vi "Item History.vi"(11 "reference in":T1) -> (3 "reference out":T1)   [LabVIEW 2016]
uses:
  Control/State machine.ctl
  <vilib>/Utility/miscctls.llb/LVPointTypeDef.ctl
  <vilib>/addons/database/NI_Database_API.lvlib
  <vilib>/addons/database/Recordset.llb/Rec Fetch Recordset Data (R).vi
  <vilib>/addons/database/Recordset.llb/Rec Destroy - Connection.vi
  <vilib>/addons/database/Connection.llb/Conn Execute.vi
  <vilib>/addons/database/_DB Variant To Data/Database Variant To Data.xnode
  <vilib>/Utility/miscctls.llb/LVRowAndColumnUnsignedTypeDef.ctl
  <vilib>/addons/database/Connection.llb/DB Tools Open Connec (Path).vi
  <vilib>/addons/database/Connection.llb/Conn ObjectReference.ctl
panel:
  in  "Sort data":string[][](array[string])
  in  "Mode":bool=TRUE
  in  "Stock":string
  in  "Location":string
  in  "Lot Size":string
  in  "Maker":string
  in  "Part Name":string
  in  "Part No.":string
  in  "Product":string
  in  "Select Month":timestamp format="%<%d/%m/%Y>T"
  in  "Item Code":string(combo)
  out "Table":string[][](table)
  # "ITEM HISTORY"
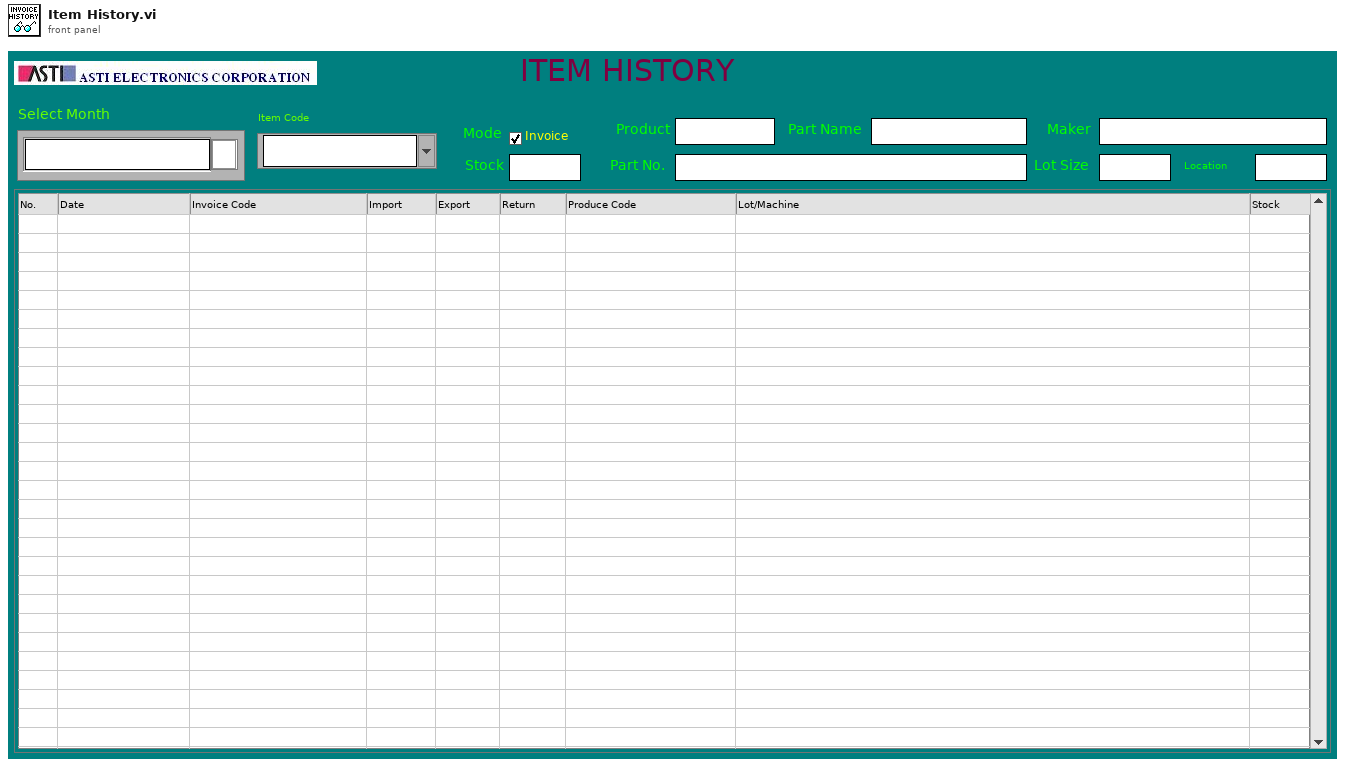
[diagram p1: front panel]
types:
  T1 = typedef "NI_Database_API.lvlib/Conn ObjectReference.ctl" = refnum<k1>
  T2 = typedef "LVPointTypeDef.ctl" = cluster{"Horizontal":i16, "Vertical":i16}
  T3 = typedef "State machine.ctl" = enum16{"Licence check", "Initial", "Log in", "Creat Config file", "Network setting", "Creat database 1", "Creat database 2", "Creat database 3", "Transfer", "Begin", "Exit"}
  T4 = typedef "LVRowAndColumnUnsignedTypeDef.ctl" = cluster{"Row":u32, "Column":u32}
  T5 = typedef "NI_Database_API.lvlib/Rec ObjectReference.ctl" = refnum<k1>
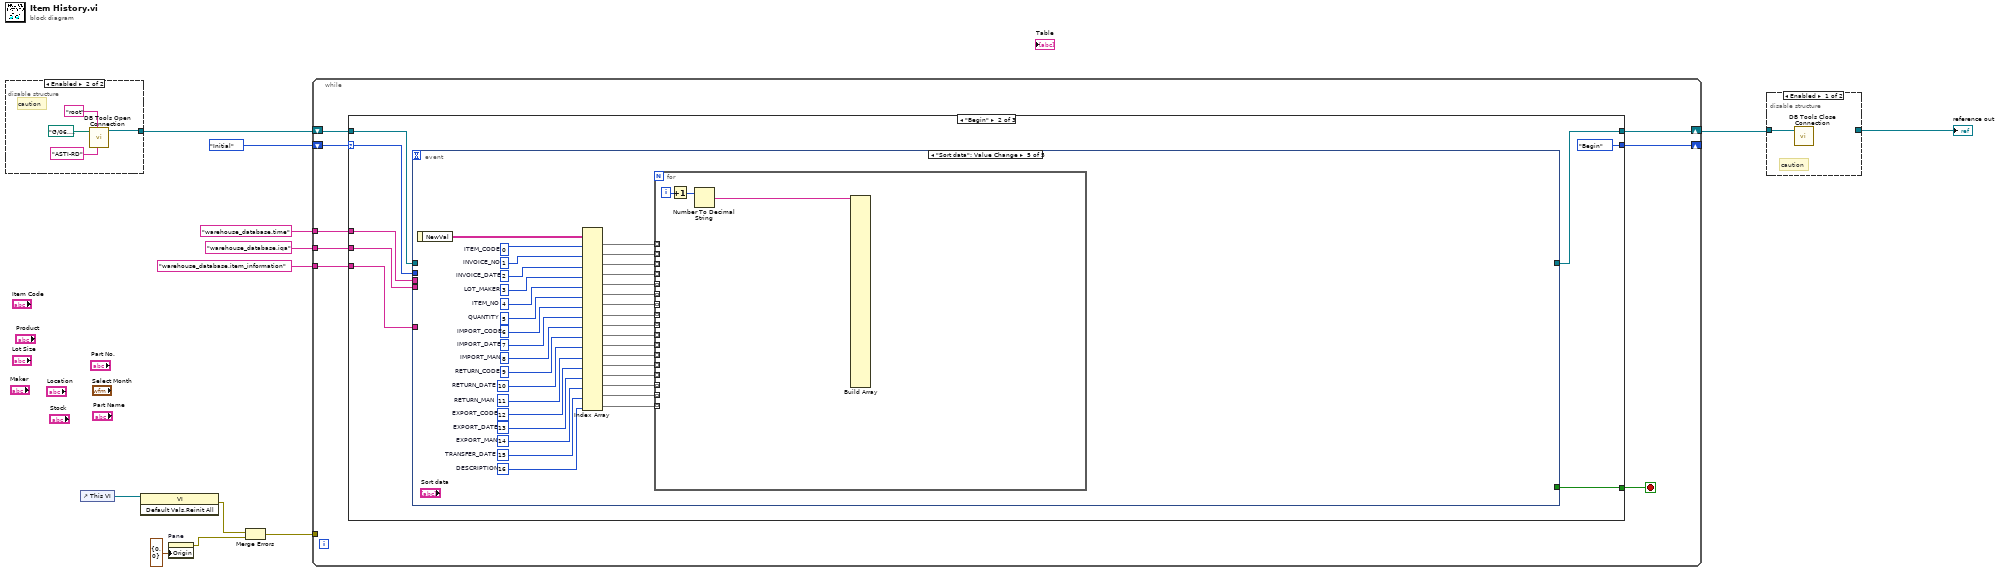
[diagram p0: block diagram]
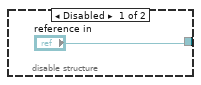
[diagram p3: hidden frame]
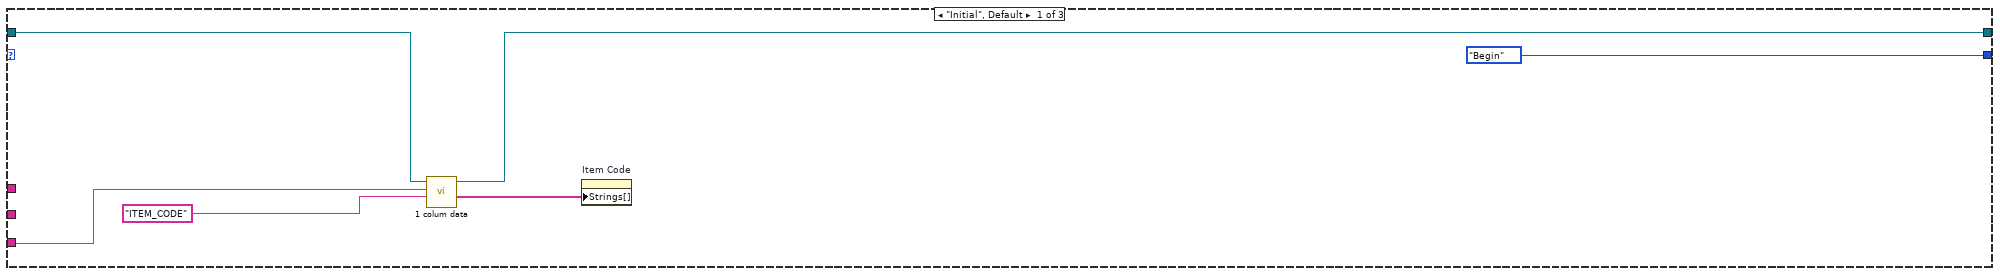
[diagram p4: hidden frame]
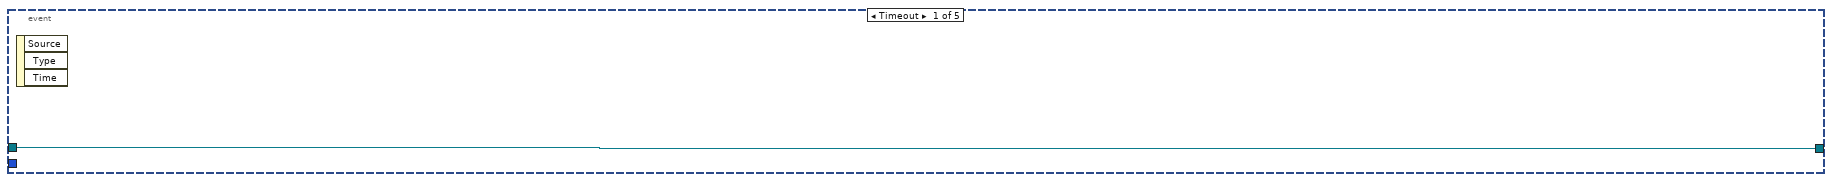
[diagram p5: hidden frame]
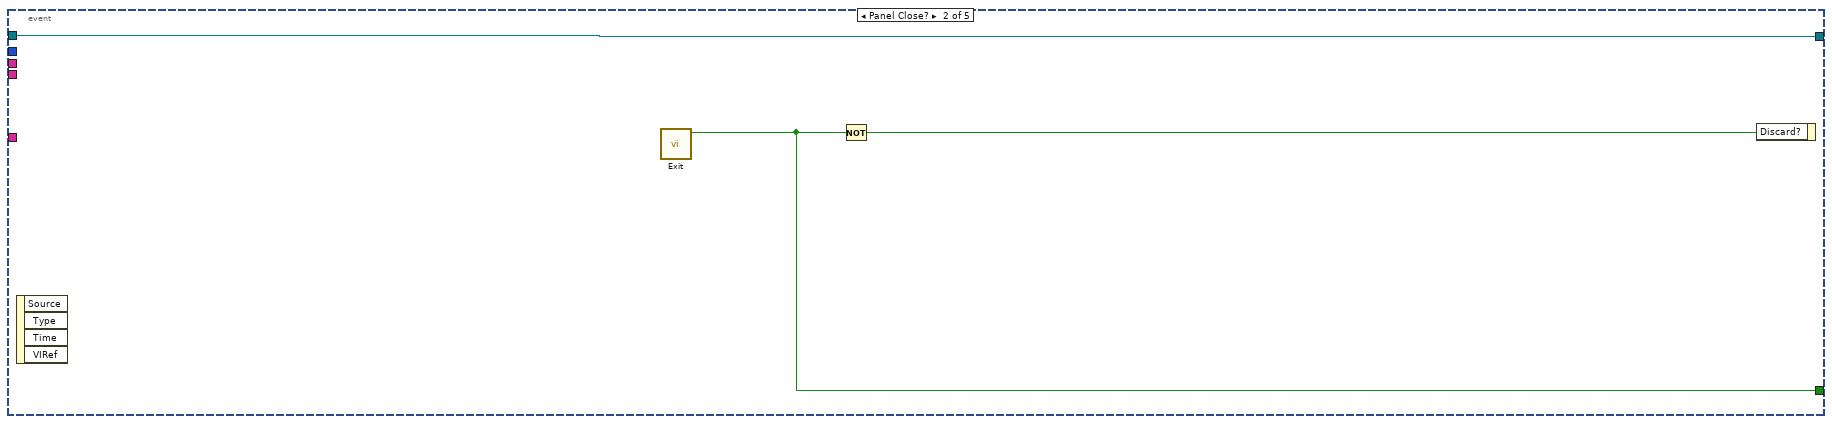
[diagram p6: hidden frame]
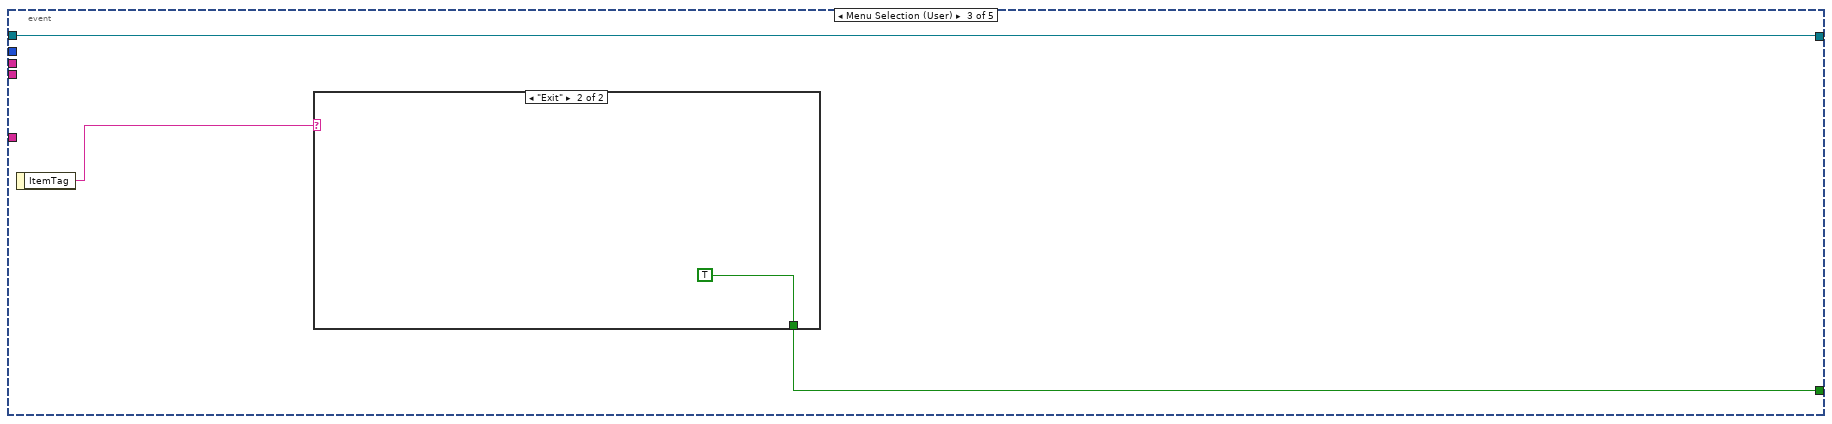
[diagram p7: hidden frame]
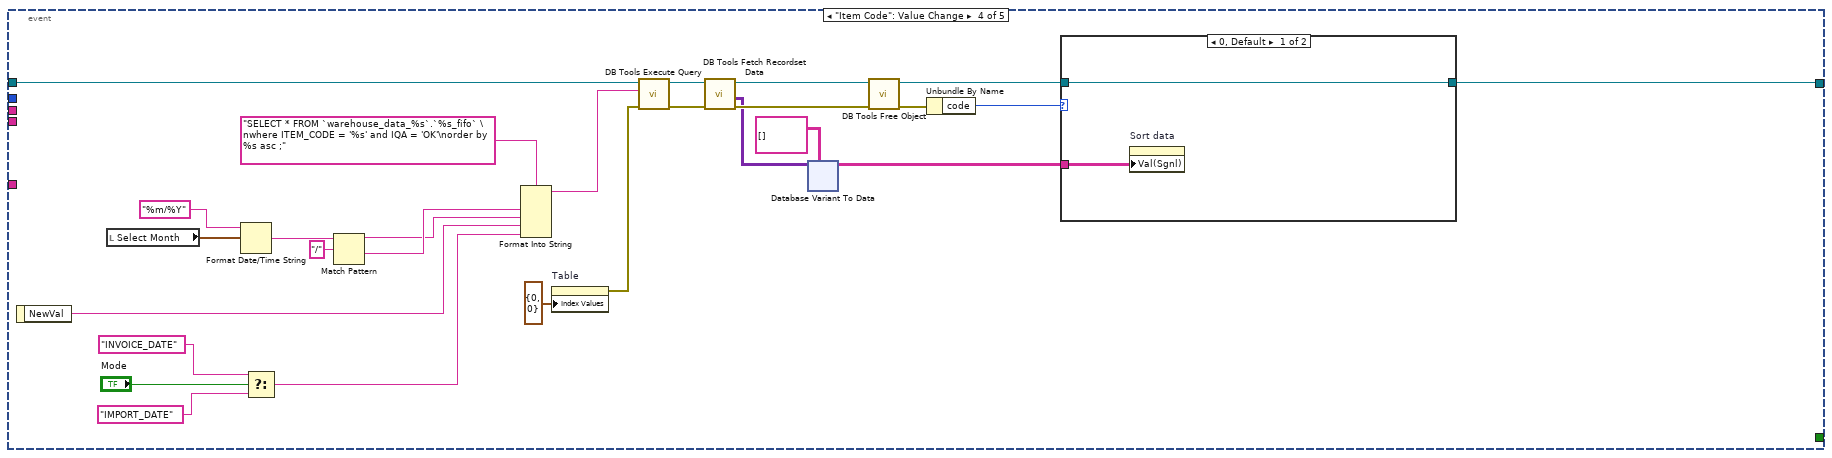
[diagram p9: hidden frame]
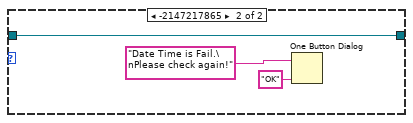
[diagram p10: hidden frame]
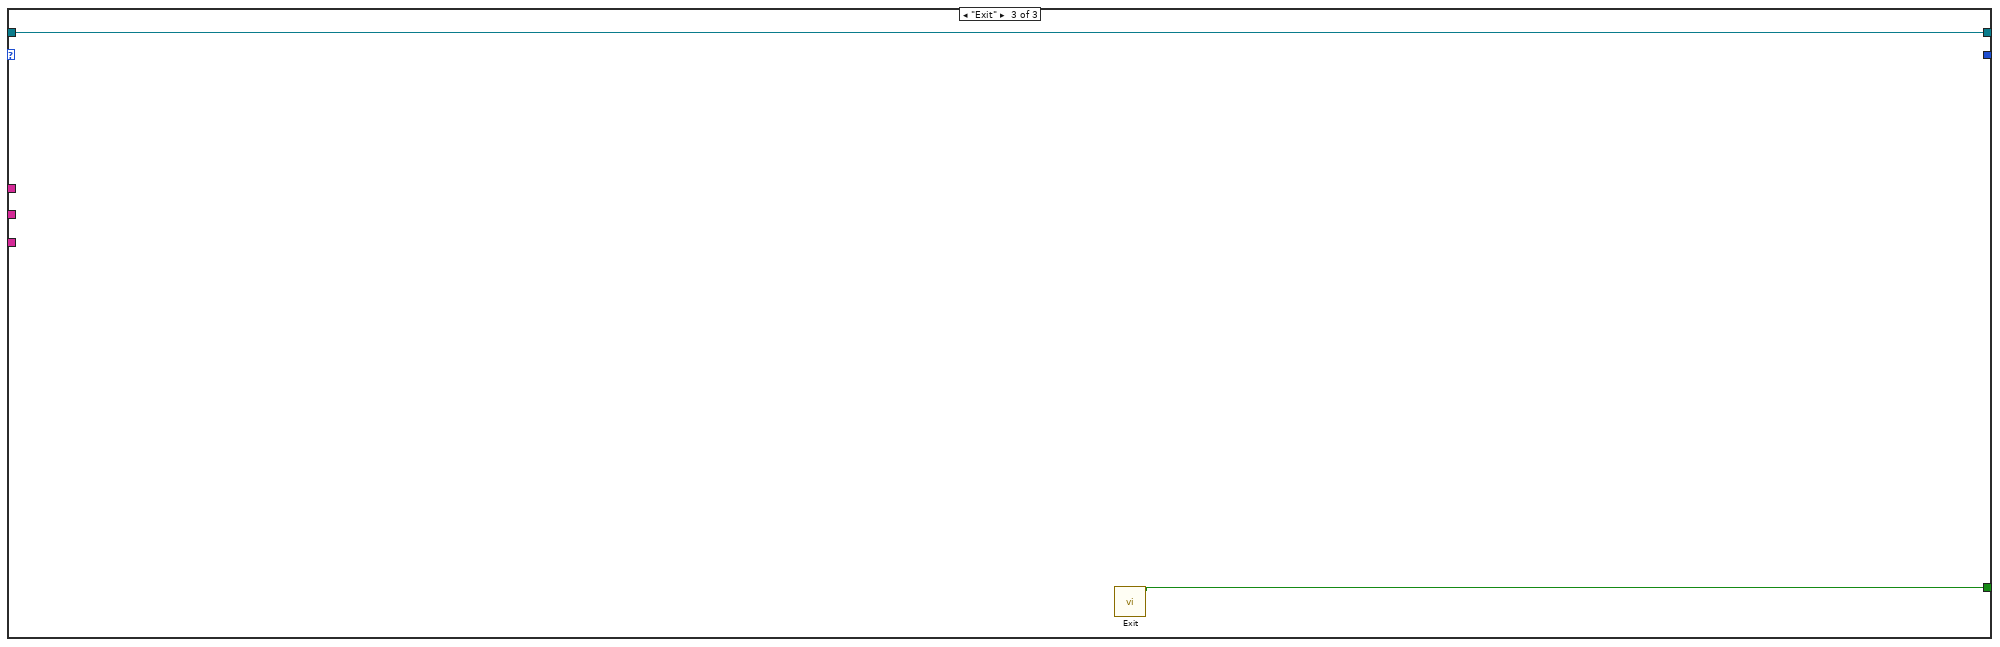
[diagram p11: hidden frame]
diagram:
  n1 = disable-structure shown="Enabled" {
    disable-tunnel: ["reference in" w17] -> w3
    frame Disabled {
    }
    frame Enabled {
      # "caution"
      n2 = call-poly <vilib>:"DB Tools Open Connection.vi"("password"="ASTI-RD", "userID"="root", "connection information"=path "G:/06. Data/Data/05. AEC/07. New Storage Management/Setting/Database local.dsn") -> ("connection reference"=w17:T1)  [unwired: 5 in, 1 out]
    }
  }
  n3 = control-ref of="This VI"() -> (w11:refnum<vi>)
  n4 = invoke class="VI" method="Default Vals.Reinit All"(reference=w11) -> (error out=w9:errorcluster)  [unwired: 2 in, 2 out]
  n5 = property on="Pane" class="Pane"("Origin"=T2 {"Horizontal"=0, "Vertical"=0}) -> (error out=w8:errorcluster)  [unwired: 2 in, 1 out]
  n6 = Merge Errors(w9, w8) -> (w7:errorcluster)
  n7 = while {
    shift-right: [w23] -> _
    shift-left: State_machine."Initial" ("Enum") -> [w24]
    shift-right: [w22] -> w2
    shift-left: w3 -> [w21]
    tunnel: w7 -> [_]
    tunnel: "warehouse_database.time" ("table") -> [w20]
    tunnel: "warehouse_database.iqa" ("table") -> [w19]
    tunnel: "warehouse_database.item_information" -> [w18]
    stop <- w25 stop-if-true
    n8 = case shown="\"Begin\"" w24 {
      selector: w24 -> [_ w36 _]
      tunnel: [_ w39 w162] -> w25
      tunnel: [State_machine."Begin" ("Enum") State_machine."Begin" ("Enum") _] -> w23
      tunnel: [w29 w37 w163] -> w22
      tunnel: w21 -> [w30 w38 w163]
      tunnel: w20 -> [_ w34 _]
      tunnel: w19 -> [_ w33 _]
      tunnel: w18 -> [w26 w32 _]
      frame "Initial", Default {
        n9 = call "1 colum data.vi"("column"="ITEM_CODE" ("String"), "table"=w26, "Refnum in"=w30) -> ("data"=w27:string[], "Refnum out"=w29:T1)  [unwired: 6 in, 1 out]
        n10 = property on="Item Code" class="CmbBox"("Strings[]"=w27) -> ()  [unwired: 2 in, 2 out]
      }
      frame "Begin" {
        n11 = event shown="[4] \"Sort data\": Value Change" {
          selector: _ -> [_ _ _ _ _]
          dyn-events: _ -> [_ _ _ _ _]
          timeout: _ -> [_ _ _ _ _]
          tunnel: [_ w43 w45 _ _] -> w39
          tunnel: w38 -> [w40 w41 w44 w74 _]
          tunnel: [w40 w41 w44 w55 _] -> w37
          tunnel: w36 -> [_ _ _ _ _]
          tunnel: w34 -> [_ _ _ _ _]
          tunnel: w33 -> [_ _ _ _ _]
          tunnel: w32 -> [_ _ _ _ _]
          event Timeout {
            n12 = event-data() -> ()  [unwired: 1 in, 3 out]
          }
          event Panel Close? {
            n13 = event-data() -> ()  [unwired: 1 in, 4 out]
            n14 = call "Exit.vi"() -> ("T button?"=w43:bool)  [unwired: 11 in]
            n15 = Not(x=w43) -> (.not. x?=w42:bool)
            n16 = event-data("Discard?"=w42) -> ()  [unwired: 1 in, 1 out]
          }
          event Menu Selection (User) {
            n17 = event-data() -> ("ItemTag"=w46:string)  [unwired: 1 in]
            n18 = case shown="\"Exit\"" w46 {
              tunnel: [_ TRUE] -> w45
              frame "False", Default {
              }
              frame "Exit" {
              }
            }
          }
          event "Item Code": Value Change {
            n19 = event-data() -> ("NewVal"=w61:string)  [unwired: 1 in]
            n20 = local read "Select Month"() -> (w69:timestamp)
            n21 = Format Date/Time String(time format string (%c)="%m/%Y", seconds (now)=w69) -> (date/time string=w67:string)  [unwired: 1 in]
            n22 = Select(t="INVOICE_DATE", s="Mode", f="IMPORT_DATE") -> (s? t:f=w51:string)
            n23 = Match Pattern(string=w67, regular expression="/") -> (before substring=w62:string, after substring=w63:string)  [unwired: 1 in, 2 out]
            n24 = Format Into String(format string="SELECT * FROM `warehouse_data_%s`.`%s_fifo` \nwhere ITEM_CODE = '%s' and IQA = 'OK'\norder by %s asc ;", w63, w62, w61, w51) -> (resulting string=w64:string)  [unwired: 2 in, 1 out]
            n25 = property on="Table" class="Tbl (strict)"("Index Values"=T4 {"Row"=0, "Column"=0}) -> (error out=w53:errorcluster)  [unwired: 2 in, 1 out]
            n26 = call-poly <vilib>:"DB Tools Execute Query.vi"("error in (no error)"=w53, "SQL query"=w64, "connection reference"=w74) -> ("error out"=w71:errorcluster, "recordset reference"=w73:T5)  [unwired: 5 in]
            n27 = call-poly <vilib>:"DB Tools Fetch Recordset Data.vi"("error in (no error)"=w71, "recordset reference"=w73) -> ("error out"=w70:errorcluster, "recordset data"=w60:variant[][], "recordset reference out"=w72:T5)  [unwired: 3 in]
            n28 = xnode "Database Variant To Data"("database variant"=w60, "type"=string[][] []) -> ("data"=w48:string[][])  [unwired: 1 in, 1 out]
            n29 = call-poly <vilib>:"DB Tools Free Object.vi"("error in (no error)"=w70, "recordset reference"=w72) -> ("error out"=w58:errorcluster, "connection reference"=w56:T1)  [unwired: 8 in]
            n30 = Unbundle By Name(w58) -> ("code"=w57:i32)
            n31 = case shown="0, Default" w57 {
              tunnel: [w76 w79] -> w55
              tunnel: w56 -> [w76 w79]
              tunnel: w48 -> [w75 _]
              frame 0, Default {
                n32 = property on="Sort data" class="Arr (strict)"("Val(Sgnl)"=w75) -> ()  [unwired: 2 in, 2 out]
              }
              frame -2147217865 {
                n33 = One Button Dialog(message="Date Time is Fail.\nPlease check again!", button name ("OK")="OK") -> ()  [unwired: 1 out]
              }
            }
          }
          event "Sort data": Value Change {
            w141 = 16  # DESCRIPTION
            w142 = 15  # TRANSFER_DATE
            w143 = 14  # EXPORT_MAN
            w144 = 13  # EXPORT_DATE
            w145 = 12  # EXPORT_CODE
            w146 = 11  # RETURN_MAN
            w147 = 10  # RETURN_DATE
            w148 = 9  # RETURN_CODE
            w149 = 8  # IMPORT_MAN
            w150 = 7  # IMPORT_DATE
            w151 = 6  # IMPORT_CODE
            w152 = 5  # QUANTITY
            w153 = 4  # ITEM_NO
            w154 = 3  # LOT_MAKER
            w155 = 2  # INVOICE_DATE
            w156 = 1  # INVOICE_NO
            w157 = 0  # ITEM_CODE
            n34 = event-data() -> ("NewVal"=w158:string[][])  [unwired: 1 in]
            n35 = Index Array(array=w158, index (col) #1=w157, index (col) #2=w156, index (col) #3=w155, index (col) #4=w154, index (col) #5=w153, index (col) #6=w152, index (col) #7=w151, index (col) #8=w150, index (col) #9=w149, index (col) #10=w148, index (col) #11=w147, index (col) #12=w146, index (col) #13=w145, index (col) #14=w144, index (col) #15=w143, index (col) #16=w142, index (col) #17=w141) -> (element #1=w140:string[], element #2=w139:string[], element #3=w138:string[], element #4=w137:string[], element #5=w136:string[], element #6=w135:string[], element #7=w134:string[], element #8=w133:string[], element #9=w132:string[], element #10=w131:string[], element #11=w130:string[], element #12=w129:string[], element #13=w128:string[], element #14=w127:string[], element #15=w126:string[], element #16=w125:string[], element #17=w124:string[])  [unwired: 17 in]
            n36 = for {
              tunnel: w140 -> [_] mode=indexing
              tunnel: w139 -> [_] mode=indexing
              tunnel: w138 -> [_] mode=indexing
              tunnel: w137 -> [_] mode=indexing
              tunnel: w136 -> [_] mode=indexing
              tunnel: w135 -> [_] mode=indexing
              tunnel: w134 -> [_] mode=indexing
              tunnel: w133 -> [_] mode=indexing
              tunnel: w132 -> [_] mode=indexing
              tunnel: w131 -> [_] mode=indexing
              tunnel: w130 -> [_] mode=indexing
              tunnel: w129 -> [_] mode=indexing
              tunnel: w128 -> [_] mode=indexing
              tunnel: w127 -> [_] mode=indexing
              tunnel: w126 -> [_] mode=indexing
              tunnel: w125 -> [_] mode=indexing
              tunnel: w124 -> [_] mode=indexing
              i -> [w161]
              n37 = Increment(x=w161) -> (x+1=w160:i32)
              n38 = Number To Decimal String(number=w160) -> (decimal integer string=w159:string)  [unwired: 1 in]
              n39 = Build Array(w159) -> ()  [unwired: 37 in, 1 out]
            }
          }
        }
      }
      frame "Exit" {
        n40 = call "Exit.vi"() -> ("T button?"=w162:bool)  [unwired: 11 in]
      }
    }
  }
  n41 = disable-structure shown="Enabled" {
    disable-tunnel: w2 -> [w164 w165]
    disable-tunnel: [_ w165] -> w1
    frame Enabled {
      # "caution"
      n42 = call <vilib>:"DB Tools Close Connection.vi"("connection reference"=w164) -> ()  [unwired: 6 in, 1 out]
    }
    frame Disabled {
    }
  }
  "reference out" <- w1
